vi "Tosca-Process AI Double Click.vi"(0 "state in":T1, 1 "Legend":refnum<vi>, 7 "Row":i32) -> (4 "state out":T1)   [LabVIEW 2020]
uses:
  Typedefs/Tosca-AI UI State.ctl
  Typedefs/Tosca-AI Plot Properties.ctl
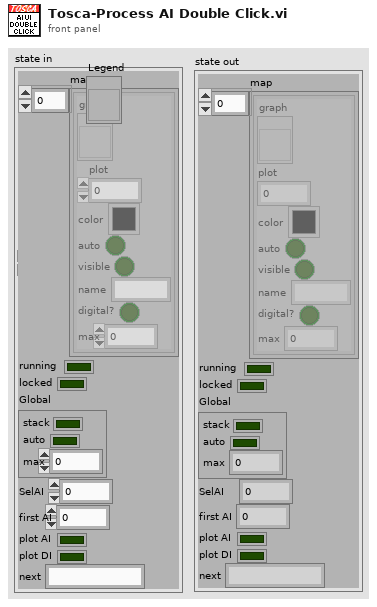
[diagram p1: front panel]
types:
  T1 = typedef "Tosca-AI UI State.ctl" = cluster{"map":T2[], "running":bool, "locked":bool, "Global":cluster{"stack":bool, "auto":bool, "max":dbl}, "SelAI":i32, "first AI":i32, "plot AI":bool, "plot DI":bool, "next":string}
  T2 = typedef "Tosca-AI Plot Properties.ctl" = cluster{"graph":refnum<vi>, "plot":i32, "color":u32, "auto":bool, "visible":bool, "name":string, "digital?":bool, "max":dbl}
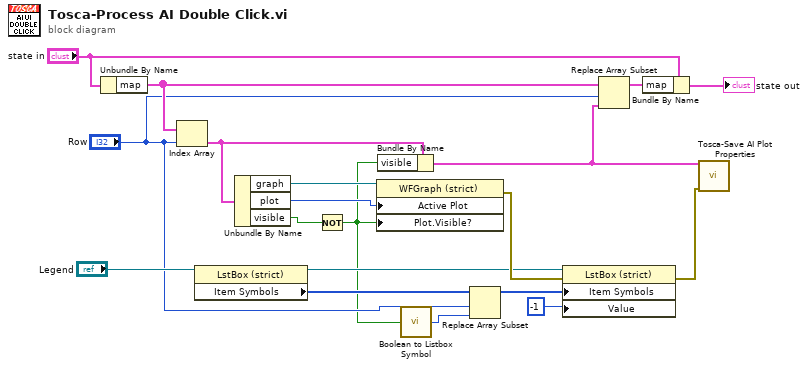
[diagram p0: block diagram]
diagram:
  n1 = Unbundle By Name("state in") -> ("map"=w16:T2[])
  n2 = Index Array(array=w16, index="Row") -> (element=w17:T2)
  n3 = property class="LstBox (strict)"(reference="Legend") -> (reference out=w6:refnum<vi>, "Item Symbols"=w5:i32[])  [unwired: 1 in, 1 out]
  n4 = Unbundle By Name(w17) -> ("graph"=w19:refnum<vi>, "plot"=w18:i32, "visible"=w8:bool)
  n5 = Not(x=w8) -> (.not. x?=w1:bool)
  n6 = property class="WFGraph (strict)"(reference=w19, "Active Plot"=w18, "Plot.Visible?"=w1) -> (error out=w12:errorcluster)  [unwired: 1 in, 1 out]
  n7 = Bundle By Name(cluster=w17, "visible"=w1) -> (w10:T2)
  n8 = call "Boolean to Listbox Symbol.vi"("Boolean"=w1) -> ("Symbol"=w2:i32)  [unwired: 14 in]
  n9 = Replace Array Subset(array=w5, new element=w2, index="Row") -> (w4:i32[])
  n10 = property class="LstBox (strict)"(reference=w6, error in=w12, "Item Symbols"=w4, "Value"=-1) -> (error out=w9:errorcluster)  [unwired: 1 out]
  n11 = Replace Array Subset(array=w16, new element=w10, index="Row") -> (w13:T2[])
  n12 = Bundle By Name(cluster="state in", "map"=w13) -> (→"state out":T1)
  n13 = call "Tosca-Save AI Plot Properties.vi"("plot"=w10, "error in (no error)"=w9) -> ()  [unwired: 14 in]
